vi "02.1 Parallel Loops.vi"() -> ()   [LabVIEW 2019]
uses:
  <extravilib>/ChannelInstances/Stream-dbl/EndpointRead.vi
  <extravilib>/ChannelInstances/Stream-dbl/Endpoint.vi
  <extravilib>/ChannelInstances/Stream-dbl/Instantiate.vi
  <extravilib>/ChannelInstances/Stream-dbl/)Channel.vi
  <resource>/ChannelSupport/_ChannelSupport/WaitIfNeeded.vi
  <extravilib>/ChannelInstances/Stream-dbl.lvlib
panel:
  out "Chart B":dbl(graph)
  out "Chart A":dbl(graph)
  in  "Stop Producer Loop 3":bool
  in  "Stop Consumer Loop 2":bool
  out "Producer iterations 2":i32
  out "Producer data 2":dbl
  in  "Stop Producer Loop 2":bool
  out "Consumer data 2":dbl
  out "Consumer iterations 2":i32
  in  "Stop Consumer Loop":bool
  out "Consumer iterations":i32
  out "Consumer data":dbl
  in  "Stop Producer Loop":bool
  out "Producer data":dbl
  out "Producer iterations":i32
  # "PRODUCER LOOP"
  # "CONSUMER LOOP"
  # "Using Channel wire"
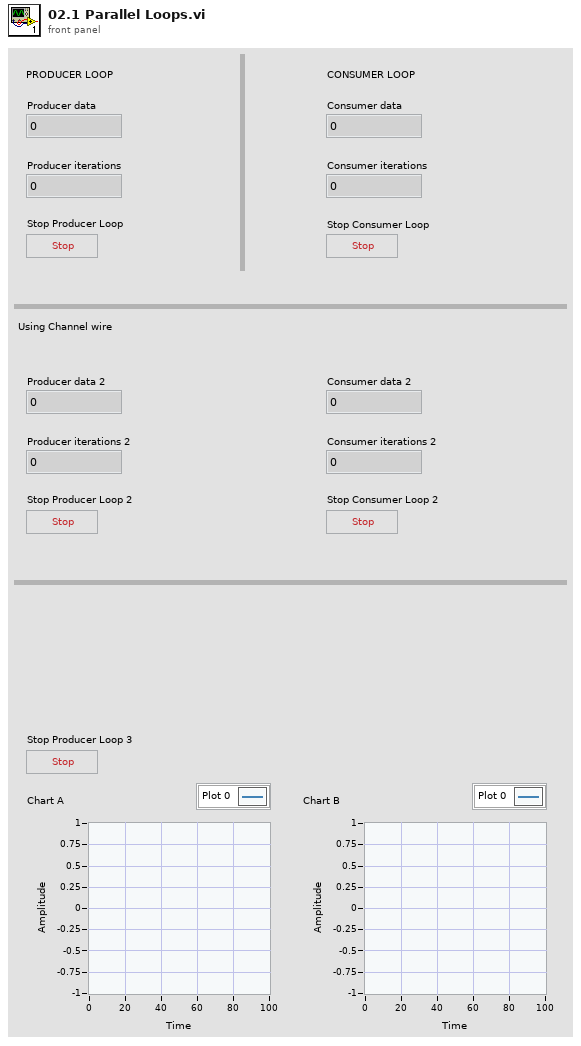
[diagram p1: front panel]
types:
  T1 = typedef "Stream-dbl.lvlib/)Channel.ctl" = refnum<queue>
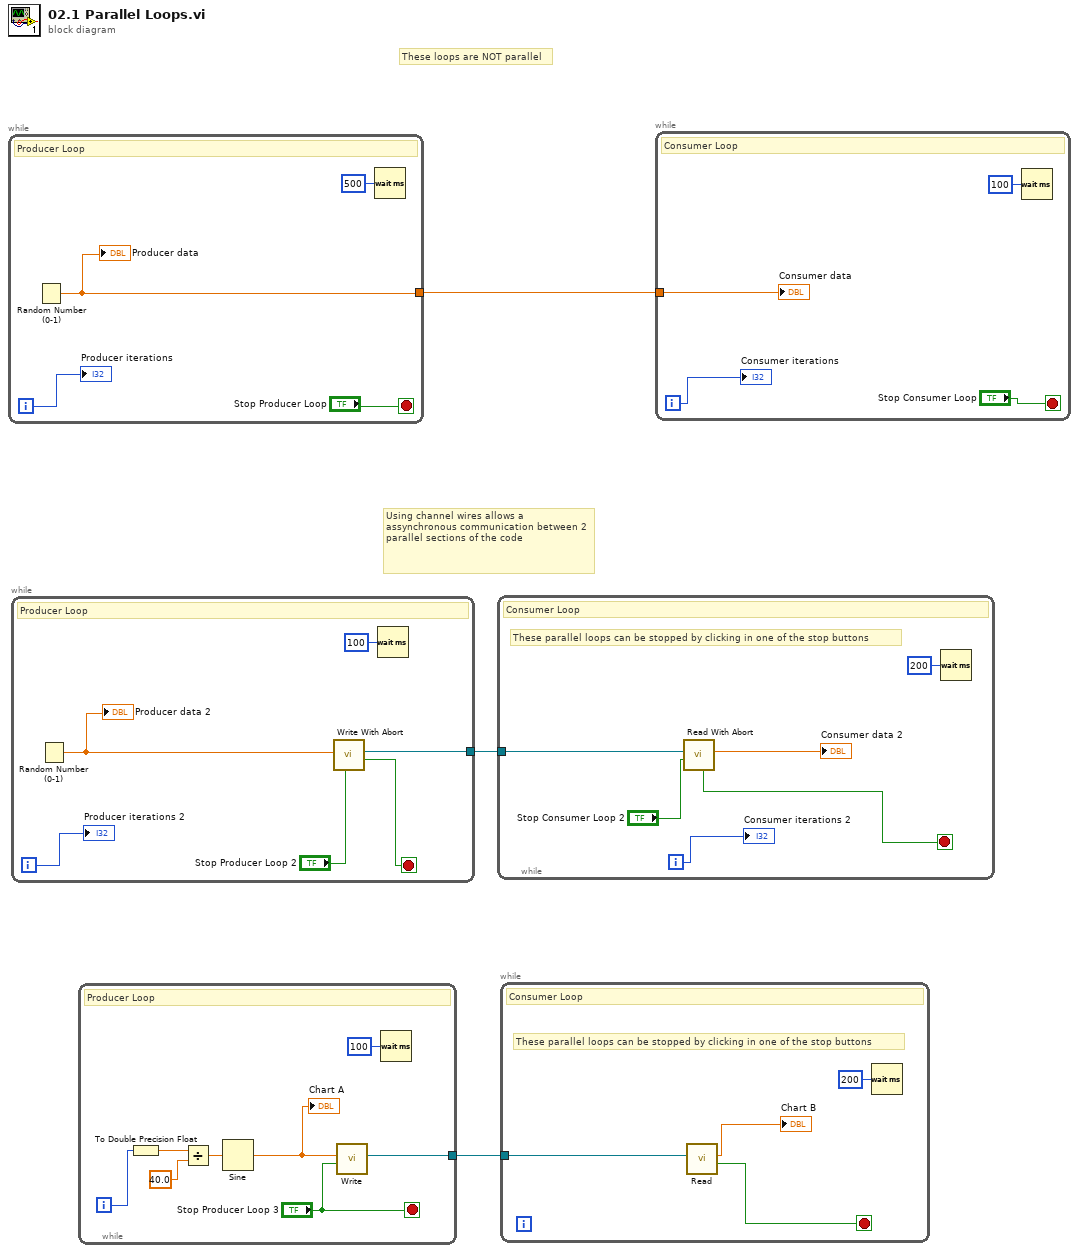
[diagram p0: block diagram]
diagram:
  # "Using channel wires allows a assynchronous communication between 2 parallel sections of the code"
  # "These loops are NOT parallel"
  n1 = while {
    tunnel: [w6] -> w3
    i -> [w5]
    stop <- "Stop Producer Loop" stop-if-true
    # "Producer Loop"
    n2 = Random Number (0-1)() -> (number: 0 to 1=w6:dbl)
    "Producer data" <- w6
    n3 = Wait (ms)(milliseconds to wait=u32 500) -> ()  [unwired: 1 out]
    "Producer iterations" <- w5
  }
  n4 = while {
    tunnel: [w10] -> w2
    i -> [w11]
    stop <- w8 stop-if-true
    # "Producer Loop"
    n5 = Random Number (0-1)() -> (number: 0 to 1=w12:dbl)
    "Producer data 2" <- w12
    n6 = call <extravilib>:"Write With Abort.vi"("abort"="Stop Producer Loop 2", "element"=w12) -> ("aborted?"=w8:bool, "channel"=w10:T1)  [unwired: 6 in, 2 out]
    n7 = Wait (ms)(milliseconds to wait=u32 100) -> ()  [unwired: 1 out]
    "Producer iterations 2" <- w11
  }
  n8 = while {
    tunnel: [w20] -> w1
    i -> [w14]
    stop <- "Stop Producer Loop 3" stop-if-true
    # "Producer Loop"
    n9 = To Double Precision Float(number=w14) -> (double precision float=w15:dbl)
    n10 = Divide(x=w15, y=40.0) -> (x/y=w17:dbl)
    n11 = Sine(x=w17) -> (sin(x)=w18:dbl)
    "Chart A" <- w18
    n12 = call <extravilib>:"Write.vi"("last element? (F)"="Stop Producer Loop 3", "element"=w18) -> ("channel"=w20:T1)  [unwired: 7 in, 2 out]
    n13 = Wait (ms)(milliseconds to wait=u32 100) -> ()  [unwired: 1 out]
  }
  n14 = while {
    tunnel: w2 -> [w25]
    i -> [w26]
    stop <- w23 stop-if-true
    # "These parallel loops can be stopped by clicking in one of the stop buttons"
    # "Consumer Loop"
    n15 = call <extravilib>:"Read With Abort.vi"("abort"="Stop Consumer Loop 2", "channel"=w25) -> ("element"=→"Consumer data 2":dbl, "aborted?"=w23:bool)  [unwired: 4 in, 4 out]
    n16 = Wait (ms)(milliseconds to wait=u32 200) -> ()  [unwired: 1 out]
    "Consumer iterations 2" <- w26
  }
  n17 = while {
    tunnel: w1 -> [w30]
    stop <- w29 stop-if-true
    # "These parallel loops can be stopped by clicking in one of the stop buttons"
    # "Consumer Loop"
    n18 = call <extravilib>:"Read.vi"("channel"=w30) -> ("last element?"=w29:bool, "element"=→"Chart B":dbl)  [unwired: 6 in, 3 out]
    n19 = Wait (ms)(milliseconds to wait=u32 200) -> ()  [unwired: 1 out]
  }
  n20 = while {
    tunnel: w3 -> [w34]
    i -> [w33]
    stop <- "Stop Consumer Loop" stop-if-true
    # "Consumer Loop"
    n21 = Wait (ms)(milliseconds to wait=u32 100) -> ()  [unwired: 1 out]
    "Consumer data" <- w34
    "Consumer iterations" <- w33
  }
